vi "EncodeBase64.vi"(10 "string":string) -> (2 "base64 string":string)   [LabVIEW 2014]
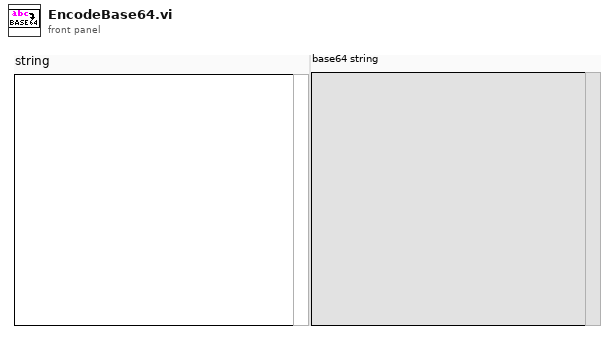
[diagram p1: front panel]
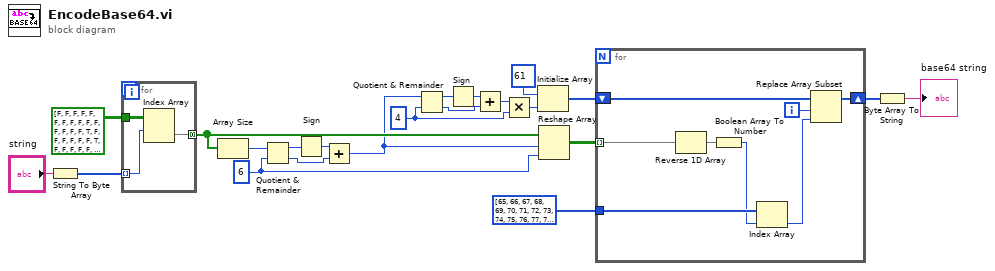
[diagram p0: block diagram]
diagram:
  w2 = 4 ("y")
  w19 = 6 ("y")
  n1 = String To Byte Array(string="string") -> (unsigned byte array=w11:u8[])
  n2 = for {
    tunnel: bool[][] [[FALSE, FALSE, FALSE, FALSE, FALSE, FALSE, FALSE, FALSE], [FALSE, FALSE, FALSE, FALSE, FALSE, FALSE, FALSE, TRUE], [FALSE, FALSE, FALSE, FALSE, FALSE, FALSE, TRUE, FALSE], [FALSE, FALSE, FALSE, FALSE, FALSE, FALSE, TRUE, TRUE], [FALSE, FALSE, FALSE, FALSE, FALSE, TRUE, FALSE, FALSE], [FALSE, FALSE, FALSE, FALSE, FALSE, TRUE, FALSE, TRUE], [FALSE, FALSE, FALSE, FALSE, FALSE, TRUE, TRUE, FALSE], [FALSE, FALSE, FALSE, FALSE, FALSE, TRUE, TRUE, TRUE], [FALSE, FALSE, FALSE, FALSE, TRUE, FALSE, FALSE, FALSE], [FALSE, FALSE, FALSE, FALSE, TRUE, FALSE, FALSE, TRUE], [FALSE, FALSE, FALSE, FALSE, TRUE, FALSE, TRUE, FALSE], [FALSE, FALSE, FALSE, FALSE, TRUE, FALSE, TRUE, TRUE], [FALSE, FALSE, FALSE, FALSE, TRUE, TRUE, FALSE, FALSE], [FALSE, FALSE, FALSE, FALSE, TRUE, TRUE, FALSE, TRUE], [FALSE, FALSE, FALSE, FALSE, TRUE, TRUE, TRUE, FALSE], [FALSE, FALSE, FALSE, FALSE, TRUE, TRUE, TRUE, TRUE], [FALSE, FALSE, FALSE, TRUE, FALSE, FALSE, FALSE, FALSE], [FALSE, FALSE, FALSE, TRUE, FALSE, FALSE, FALSE, TRUE], [FALSE, FALSE, FALSE, TRUE, FALSE, FALSE, TRUE, FALSE], [FALSE, FALSE, FALSE, TRUE, FALSE, FALSE, TRUE, TRUE], [FALSE, FALSE, FALSE, TRUE, FALSE, TRUE, FALSE, FALSE], [FALSE, FALSE, FALSE, TRUE, FALSE, TRUE, FALSE, TRUE], [FALSE, FALSE, FALSE, TRUE, FALSE, TRUE, TRUE, FALSE], [FALSE, FALSE, FALSE, TRUE, FALSE, TRUE, TRUE, TRUE], [FALSE, FALSE, FALSE, TRUE, TRUE, FALSE, FALSE, FALSE], [FALSE, FALSE, FALSE, TRUE, TRUE, FALSE, FALSE, TRUE], [FALSE, FALSE, FALSE, TRUE, TRUE, FALSE, TRUE, FALSE], [FALSE, FALSE, FALSE, TRUE, TRUE, FALSE, TRUE, TRUE], [FALSE, FALSE, FALSE, TRUE, TRUE, TRUE, FALSE, FALSE], [FALSE, FALSE, FALSE, TRUE, TRUE, TRUE, FALSE, TRUE], [FALSE, FALSE, FALSE, TRUE, TRUE, TRUE, TRUE, FALSE], [FALSE, FALSE, FALSE, TRUE, TRUE, TRUE, TRUE, TRUE], [FALSE, FALSE, TRUE, FALSE, FALSE, FALSE, FALSE, FALSE], [FALSE, FALSE, TRUE, FALSE, FALSE, FALSE, FALSE, TRUE], [FALSE, FALSE, TRUE, FALSE, FALSE, FALSE, TRUE, FALSE], [FALSE, FALSE, TRUE, FALSE, FALSE, FALSE, TRUE, TRUE], [FALSE, FALSE, TRUE, FALSE, FALSE, TRUE, FALSE, FALSE], [FALSE, FALSE, TRUE, FALSE, FALSE, TRUE, FALSE, TRUE], [FALSE, FALSE, TRUE, FALSE, FALSE, TRUE, TRUE, FALSE], [FALSE, FALSE, TRUE, FALSE, FALSE, TRUE, TRUE, TRUE], [FALSE, FALSE, TRUE, FALSE, TRUE, FALSE, FALSE, FALSE], [FALSE, FALSE, TRUE, FALSE, TRUE, FALSE, FALSE, TRUE], [FALSE, FALSE, TRUE, FALSE, TRUE, FALSE, TRUE, FALSE], [FALSE, FALSE, TRUE, FALSE, TRUE, FALSE, TRUE, TRUE], [FALSE, FALSE, TRUE, FALSE, TRUE, TRUE, FALSE, FALSE], [FALSE, FALSE, TRUE, FALSE, TRUE, TRUE, FALSE, TRUE], [FALSE, FALSE, TRUE, FALSE, TRUE, TRUE, TRUE, FALSE], [FALSE, FALSE, TRUE, FALSE, TRUE, TRUE, TRUE, TRUE], [FALSE, FALSE, TRUE, TRUE, FALSE, FALSE, FALSE, FALSE], [FALSE, FALSE, TRUE, TRUE, FALSE, FALSE, FALSE, TRUE], [FALSE, FALSE, TRUE, TRUE, FALSE, FALSE, TRUE, FALSE], [FALSE, FALSE, TRUE, TRUE, FALSE, FALSE, TRUE, TRUE], [FALSE, FALSE, TRUE, TRUE, FALSE, TRUE, FALSE, FALSE], [FALSE, FALSE, TRUE, TRUE, FALSE, TRUE, FALSE, TRUE], [FALSE, FALSE, TRUE, TRUE, FALSE, TRUE, TRUE, FALSE], [FALSE, FALSE, TRUE, TRUE, FALSE, TRUE, TRUE, TRUE], [FALSE, FALSE, TRUE, TRUE, TRUE, FALSE, FALSE, FALSE], [FALSE, FALSE, TRUE, TRUE, TRUE, FALSE, FALSE, TRUE], [FALSE, FALSE, TRUE, TRUE, TRUE, FALSE, TRUE, FALSE], [FALSE, FALSE, TRUE, TRUE, TRUE, FALSE, TRUE, TRUE], [FALSE, FALSE, TRUE, TRUE, TRUE, TRUE, FALSE, FALSE], [FALSE, FALSE, TRUE, TRUE, TRUE, TRUE, FALSE, TRUE], [FALSE, FALSE, TRUE, TRUE, TRUE, TRUE, TRUE, FALSE], [FALSE, FALSE, TRUE, TRUE, TRUE, TRUE, TRUE, TRUE], [FALSE, TRUE, FALSE, FALSE, FALSE, FALSE, FALSE, FALSE], [FALSE, TRUE, FALSE, FALSE, FALSE, FALSE, FALSE, TRUE], [FALSE, TRUE, FALSE, FALSE, FALSE, FALSE, TRUE, FALSE], [FALSE, TRUE, FALSE, FALSE, FALSE, FALSE, TRUE, TRUE], [FALSE, TRUE, FALSE, FALSE, FALSE, TRUE, FALSE, FALSE], [FALSE, TRUE, FALSE, FALSE, FALSE, TRUE, FALSE, TRUE], [FALSE, TRUE, FALSE, FALSE, FALSE, TRUE, TRUE, FALSE], [FALSE, TRUE, FALSE, FALSE, FALSE, TRUE, TRUE, TRUE], [FALSE, TRUE, FALSE, FALSE, TRUE, FALSE, FALSE, FALSE], [FALSE, TRUE, FALSE, FALSE, TRUE, FALSE, FALSE, TRUE], [FALSE, TRUE, FALSE, FALSE, TRUE, FALSE, TRUE, FALSE], [FALSE, TRUE, FALSE, FALSE, TRUE, FALSE, TRUE, TRUE], [FALSE, TRUE, FALSE, FALSE, TRUE, TRUE, FALSE, FALSE], [FALSE, TRUE, FALSE, FALSE, TRUE, TRUE, FALSE, TRUE], [FALSE, TRUE, FALSE, FALSE, TRUE, TRUE, TRUE, FALSE], [FALSE, TRUE, FALSE, FALSE, TRUE, TRUE, TRUE, TRUE], [FALSE, TRUE, FALSE, TRUE, FALSE, FALSE, FALSE, FALSE], [FALSE, TRUE, FALSE, TRUE, FALSE, FALSE, FALSE, TRUE], [FALSE, TRUE, FALSE, TRUE, FALSE, FALSE, TRUE, FALSE], [FALSE, TRUE, FALSE, TRUE, FALSE, FALSE, TRUE, TRUE], [FALSE, TRUE, FALSE, TRUE, FALSE, TRUE, FALSE, FALSE], [FALSE, TRUE, FALSE, TRUE, FALSE, TRUE, FALSE, TRUE], [FALSE, TRUE, FALSE, TRUE, FALSE, TRUE, TRUE, FALSE], [FALSE, TRUE, FALSE, TRUE, FALSE, TRUE, TRUE, TRUE], [FALSE, TRUE, FALSE, TRUE, TRUE, FALSE, FALSE, FALSE], [FALSE, TRUE, FALSE, TRUE, TRUE, FALSE, FALSE, TRUE], [FALSE, TRUE, FALSE, TRUE, TRUE, FALSE, TRUE, FALSE], [FALSE, TRUE, FALSE, TRUE, TRUE, FALSE, TRUE, TRUE], [FALSE, TRUE, FALSE, TRUE, TRUE, TRUE, FALSE, FALSE], [FALSE, TRUE, FALSE, TRUE, TRUE, TRUE, FALSE, TRUE], [FALSE, TRUE, FALSE, TRUE, TRUE, TRUE, TRUE, FALSE], [FALSE, TRUE, FALSE, TRUE, TRUE, TRUE, TRUE, TRUE], [FALSE, TRUE, TRUE, FALSE, FALSE, FALSE, FALSE, FALSE], [FALSE, TRUE, TRUE, FALSE, FALSE, FALSE, FALSE, TRUE], [FALSE, TRUE, TRUE, FALSE, FALSE, FALSE, TRUE, FALSE], [FALSE, TRUE, TRUE, FALSE, FALSE, FALSE, TRUE, TRUE], [FALSE, TRUE, TRUE, FALSE, FALSE, TRUE, FALSE, FALSE], [FALSE, TRUE, TRUE, FALSE, FALSE, TRUE, FALSE, TRUE], [FALSE, TRUE, TRUE, FALSE, FALSE, TRUE, TRUE, FALSE], [FALSE, TRUE, TRUE, FALSE, FALSE, TRUE, TRUE, TRUE], [FALSE, TRUE, TRUE, FALSE, TRUE, FALSE, FALSE, FALSE], [FALSE, TRUE, TRUE, FALSE, TRUE, FALSE, FALSE, TRUE], [FALSE, TRUE, TRUE, FALSE, TRUE, FALSE, TRUE, FALSE], [FALSE, TRUE, TRUE, FALSE, TRUE, FALSE, TRUE, TRUE], [FALSE, TRUE, TRUE, FALSE, TRUE, TRUE, FALSE, FALSE], [FALSE, TRUE, TRUE, FALSE, TRUE, TRUE, FALSE, TRUE], [FALSE, TRUE, TRUE, FALSE, TRUE, TRUE, TRUE, FALSE], [FALSE, TRUE, TRUE, FALSE, TRUE, TRUE, TRUE, TRUE], [FALSE, TRUE, TRUE, TRUE, FALSE, FALSE, FALSE, FALSE], [FALSE, TRUE, TRUE, TRUE, FALSE, FALSE, FALSE, TRUE], [FALSE, TRUE, TRUE, TRUE, FALSE, FALSE, TRUE, FALSE], [FALSE, TRUE, TRUE, TRUE, FALSE, FALSE, TRUE, TRUE], [FALSE, TRUE, TRUE, TRUE, FALSE, TRUE, FALSE, FALSE], [FALSE, TRUE, TRUE, TRUE, FALSE, TRUE, FALSE, TRUE], [FALSE, TRUE, TRUE, TRUE, FALSE, TRUE, TRUE, FALSE], [FALSE, TRUE, TRUE, TRUE, FALSE, TRUE, TRUE, TRUE], [FALSE, TRUE, TRUE, TRUE, TRUE, FALSE, FALSE, FALSE], [FALSE, TRUE, TRUE, TRUE, TRUE, FALSE, FALSE, TRUE], [FALSE, TRUE, TRUE, TRUE, TRUE, FALSE, TRUE, FALSE], [FALSE, TRUE, TRUE, TRUE, TRUE, FALSE, TRUE, TRUE], [FALSE, TRUE, TRUE, TRUE, TRUE, TRUE, FALSE, FALSE], [FALSE, TRUE, TRUE, TRUE, TRUE, TRUE, FALSE, TRUE], [FALSE, TRUE, TRUE, TRUE, TRUE, TRUE, TRUE, FALSE], [FALSE, TRUE, TRUE, TRUE, TRUE, TRUE, TRUE, TRUE], [TRUE, FALSE, FALSE, FALSE, FALSE, FALSE, FALSE, FALSE], [TRUE, FALSE, FALSE, FALSE, FALSE, FALSE, FALSE, TRUE], [TRUE, FALSE, FALSE, FALSE, FALSE, FALSE, TRUE, FALSE], [TRUE, FALSE, FALSE, FALSE, FALSE, FALSE, TRUE, TRUE], [TRUE, FALSE, FALSE, FALSE, FALSE, TRUE, FALSE, FALSE], [TRUE, FALSE, FALSE, FALSE, FALSE, TRUE, FALSE, TRUE], [TRUE, FALSE, FALSE, FALSE, FALSE, TRUE, TRUE, FALSE], [TRUE, FALSE, FALSE, FALSE, FALSE, TRUE, TRUE, TRUE], [TRUE, FALSE, FALSE, FALSE, TRUE, FALSE, FALSE, FALSE], [TRUE, FALSE, FALSE, FALSE, TRUE, FALSE, FALSE, TRUE], [TRUE, FALSE, FALSE, FALSE, TRUE, FALSE, TRUE, FALSE], [TRUE, FALSE, FALSE, FALSE, TRUE, FALSE, TRUE, TRUE], [TRUE, FALSE, FALSE, FALSE, TRUE, TRUE, FALSE, FALSE], [TRUE, FALSE, FALSE, FALSE, TRUE, TRUE, FALSE, TRUE], [TRUE, FALSE, FALSE, FALSE, TRUE, TRUE, TRUE, FALSE], [TRUE, FALSE, FALSE, FALSE, TRUE, TRUE, TRUE, TRUE], [TRUE, FALSE, FALSE, TRUE, FALSE, FALSE, FALSE, FALSE], [TRUE, FALSE, FALSE, TRUE, FALSE, FALSE, FALSE, TRUE], [TRUE, FALSE, FALSE, TRUE, FALSE, FALSE, TRUE, FALSE], [TRUE, FALSE, FALSE, TRUE, FALSE, FALSE, TRUE, TRUE], [TRUE, FALSE, FALSE, TRUE, FALSE, TRUE, FALSE, FALSE], [TRUE, FALSE, FALSE, TRUE, FALSE, TRUE, FALSE, TRUE], [TRUE, FALSE, FALSE, TRUE, FALSE, TRUE, TRUE, FALSE], [TRUE, FALSE, FALSE, TRUE, FALSE, TRUE, TRUE, TRUE], [TRUE, FALSE, FALSE, TRUE, TRUE, FALSE, FALSE, FALSE], [TRUE, FALSE, FALSE, TRUE, TRUE, FALSE, FALSE, TRUE], [TRUE, FALSE, FALSE, TRUE, TRUE, FALSE, TRUE, FALSE], [TRUE, FALSE, FALSE, TRUE, TRUE, FALSE, TRUE, TRUE], [TRUE, FALSE, FALSE, TRUE, TRUE, TRUE, FALSE, FALSE], [TRUE, FALSE, FALSE, TRUE, TRUE, TRUE, FALSE, TRUE], [TRUE, FALSE, FALSE, TRUE, TRUE, TRUE, TRUE, FALSE], [TRUE, FALSE, FALSE, TRUE, TRUE, TRUE, TRUE, TRUE], [TRUE, FALSE, TRUE, FALSE, FALSE, FALSE, FALSE, FALSE], [TRUE, FALSE, TRUE, FALSE, FALSE, FALSE, FALSE, TRUE], [TRUE, FALSE, TRUE, FALSE, FALSE, FALSE, TRUE, FALSE], [TRUE, FALSE, TRUE, FALSE, FALSE, FALSE, TRUE, TRUE], [TRUE, FALSE, TRUE, FALSE, FALSE, TRUE, FALSE, FALSE], [TRUE, FALSE, TRUE, FALSE, FALSE, TRUE, FALSE, TRUE], [TRUE, FALSE, TRUE, FALSE, FALSE, TRUE, TRUE, FALSE], [TRUE, FALSE, TRUE, FALSE, FALSE, TRUE, TRUE, TRUE], [TRUE, FALSE, TRUE, FALSE, TRUE, FALSE, FALSE, FALSE], [TRUE, FALSE, TRUE, FALSE, TRUE, FALSE, FALSE, TRUE], [TRUE, FALSE, TRUE, FALSE, TRUE, FALSE, TRUE, FALSE], [TRUE, FALSE, TRUE, FALSE, TRUE, FALSE, TRUE, TRUE], [TRUE, FALSE, TRUE, FALSE, TRUE, TRUE, FALSE, FALSE], [TRUE, FALSE, TRUE, FALSE, TRUE, TRUE, FALSE, TRUE], [TRUE, FALSE, TRUE, FALSE, TRUE, TRUE, TRUE, FALSE], [TRUE, FALSE, TRUE, FALSE, TRUE, TRUE, TRUE, TRUE], [TRUE, FALSE, TRUE, TRUE, FALSE, FALSE, FALSE, FALSE], [TRUE, FALSE, TRUE, TRUE, FALSE, FALSE, FALSE, TRUE], [TRUE, FALSE, TRUE, TRUE, FALSE, FALSE, TRUE, FALSE], [TRUE, FALSE, TRUE, TRUE, FALSE, FALSE, TRUE, TRUE], [TRUE, FALSE, TRUE, TRUE, FALSE, TRUE, FALSE, FALSE], [TRUE, FALSE, TRUE, TRUE, FALSE, TRUE, FALSE, TRUE], [TRUE, FALSE, TRUE, TRUE, FALSE, TRUE, TRUE, FALSE], [TRUE, FALSE, TRUE, TRUE, FALSE, TRUE, TRUE, TRUE], [TRUE, FALSE, TRUE, TRUE, TRUE, FALSE, FALSE, FALSE], [TRUE, FALSE, TRUE, TRUE, TRUE, FALSE, FALSE, TRUE], [TRUE, FALSE, TRUE, TRUE, TRUE, FALSE, TRUE, FALSE], [TRUE, FALSE, TRUE, TRUE, TRUE, FALSE, TRUE, TRUE], [TRUE, FALSE, TRUE, TRUE, TRUE, TRUE, FALSE, FALSE], [TRUE, FALSE, TRUE, TRUE, TRUE, TRUE, FALSE, TRUE], [TRUE, FALSE, TRUE, TRUE, TRUE, TRUE, TRUE, FALSE], [TRUE, FALSE, TRUE, TRUE, TRUE, TRUE, TRUE, TRUE], [TRUE, TRUE, FALSE, FALSE, FALSE, FALSE, FALSE, FALSE], [TRUE, TRUE, FALSE, FALSE, FALSE, FALSE, FALSE, TRUE], [TRUE, TRUE, FALSE, FALSE, FALSE, FALSE, TRUE, FALSE], [TRUE, TRUE, FALSE, FALSE, FALSE, FALSE, TRUE, TRUE], [TRUE, TRUE, FALSE, FALSE, FALSE, TRUE, FALSE, FALSE], [TRUE, TRUE, FALSE, FALSE, FALSE, TRUE, FALSE, TRUE], [TRUE, TRUE, FALSE, FALSE, FALSE, TRUE, TRUE, FALSE], [TRUE, TRUE, FALSE, FALSE, FALSE, TRUE, TRUE, TRUE], [TRUE, TRUE, FALSE, FALSE, TRUE, FALSE, FALSE, FALSE], [TRUE, TRUE, FALSE, FALSE, TRUE, FALSE, FALSE, TRUE], [TRUE, TRUE, FALSE, FALSE, TRUE, FALSE, TRUE, FALSE], [TRUE, TRUE, FALSE, FALSE, TRUE, FALSE, TRUE, TRUE], [TRUE, TRUE, FALSE, FALSE, TRUE, TRUE, FALSE, FALSE], [TRUE, TRUE, FALSE, FALSE, TRUE, TRUE, FALSE, TRUE], [TRUE, TRUE, FALSE, FALSE, TRUE, TRUE, TRUE, FALSE], [TRUE, TRUE, FALSE, FALSE, TRUE, TRUE, TRUE, TRUE], [TRUE, TRUE, FALSE, TRUE, FALSE, FALSE, FALSE, FALSE], [TRUE, TRUE, FALSE, TRUE, FALSE, FALSE, FALSE, TRUE], [TRUE, TRUE, FALSE, TRUE, FALSE, FALSE, TRUE, FALSE], [TRUE, TRUE, FALSE, TRUE, FALSE, FALSE, TRUE, TRUE], [TRUE, TRUE, FALSE, TRUE, FALSE, TRUE, FALSE, FALSE], [TRUE, TRUE, FALSE, TRUE, FALSE, TRUE, FALSE, TRUE], [TRUE, TRUE, FALSE, TRUE, FALSE, TRUE, TRUE, FALSE], [TRUE, TRUE, FALSE, TRUE, FALSE, TRUE, TRUE, TRUE], [TRUE, TRUE, FALSE, TRUE, TRUE, FALSE, FALSE, FALSE], [TRUE, TRUE, FALSE, TRUE, TRUE, FALSE, FALSE, TRUE], [TRUE, TRUE, FALSE, TRUE, TRUE, FALSE, TRUE, FALSE], [TRUE, TRUE, FALSE, TRUE, TRUE, FALSE, TRUE, TRUE], [TRUE, TRUE, FALSE, TRUE, TRUE, TRUE, FALSE, FALSE], [TRUE, TRUE, FALSE, TRUE, TRUE, TRUE, FALSE, TRUE], [TRUE, TRUE, FALSE, TRUE, TRUE, TRUE, TRUE, FALSE], [TRUE, TRUE, FALSE, TRUE, TRUE, TRUE, TRUE, TRUE], [TRUE, TRUE, TRUE, FALSE, FALSE, FALSE, FALSE, FALSE], [TRUE, TRUE, TRUE, FALSE, FALSE, FALSE, FALSE, TRUE], [TRUE, TRUE, TRUE, FALSE, FALSE, FALSE, TRUE, FALSE], [TRUE, TRUE, TRUE, FALSE, FALSE, FALSE, TRUE, TRUE], [TRUE, TRUE, TRUE, FALSE, FALSE, TRUE, FALSE, FALSE], [TRUE, TRUE, TRUE, FALSE, FALSE, TRUE, FALSE, TRUE], [TRUE, TRUE, TRUE, FALSE, FALSE, TRUE, TRUE, FALSE], [TRUE, TRUE, TRUE, FALSE, FALSE, TRUE, TRUE, TRUE], [TRUE, TRUE, TRUE, FALSE, TRUE, FALSE, FALSE, FALSE], [TRUE, TRUE, TRUE, FALSE, TRUE, FALSE, FALSE, TRUE], [TRUE, TRUE, TRUE, FALSE, TRUE, FALSE, TRUE, FALSE], [TRUE, TRUE, TRUE, FALSE, TRUE, FALSE, TRUE, TRUE], [TRUE, TRUE, TRUE, FALSE, TRUE, TRUE, FALSE, FALSE], [TRUE, TRUE, TRUE, FALSE, TRUE, TRUE, FALSE, TRUE], [TRUE, TRUE, TRUE, FALSE, TRUE, TRUE, TRUE, FALSE], [TRUE, TRUE, TRUE, FALSE, TRUE, TRUE, TRUE, TRUE], [TRUE, TRUE, TRUE, TRUE, FALSE, FALSE, FALSE, FALSE], [TRUE, TRUE, TRUE, TRUE, FALSE, FALSE, FALSE, TRUE], [TRUE, TRUE, TRUE, TRUE, FALSE, FALSE, TRUE, FALSE], [TRUE, TRUE, TRUE, TRUE, FALSE, FALSE, TRUE, TRUE], [TRUE, TRUE, TRUE, TRUE, FALSE, TRUE, FALSE, FALSE], [TRUE, TRUE, TRUE, TRUE, FALSE, TRUE, FALSE, TRUE], [TRUE, TRUE, TRUE, TRUE, FALSE, TRUE, TRUE, FALSE], [TRUE, TRUE, TRUE, TRUE, FALSE, TRUE, TRUE, TRUE], [TRUE, TRUE, TRUE, TRUE, TRUE, FALSE, FALSE, FALSE], [TRUE, TRUE, TRUE, TRUE, TRUE, FALSE, FALSE, TRUE], [TRUE, TRUE, TRUE, TRUE, TRUE, FALSE, TRUE, FALSE], [TRUE, TRUE, TRUE, TRUE, TRUE, FALSE, TRUE, TRUE], [TRUE, TRUE, TRUE, TRUE, TRUE, TRUE, FALSE, FALSE], [TRUE, TRUE, TRUE, TRUE, TRUE, TRUE, FALSE, TRUE], [TRUE, TRUE, TRUE, TRUE, TRUE, TRUE, TRUE, FALSE], [TRUE, TRUE, TRUE, TRUE, TRUE, TRUE, TRUE, TRUE]] ("Array") -> [w25]
    tunnel: w11 -> [w24] mode=indexing
    tunnel: [w23] -> w20 mode=concatenating
    n3 = Index Array(array=w25, index (row)=w24) -> (element=w23:bool[])  [unwired: 1 in]
  }
  n4 = Array Size(array=w20) -> (size(s)=w21:i32)
  n5 = Quotient & Remainder(x=w21, y=w19) -> (x-y*floor(x/y)=w10:i32, floor(x/y)=w8:i32)
  n6 = Sign(1:w10) -> (0:w9:i32)
  n7 = Add(x=w9, y=w8) -> (x+y=w3:i32)
  n8 = Quotient & Remainder(x=w3, y=w2) -> (x-y*floor(x/y)=w5:i32, floor(x/y)=w1:i32)
  n9 = Sign(1:w5) -> (0:w6:i32)
  n10 = Add(x=w6, y=w1) -> (x+y=w7:i32)
  n11 = Multiply(x=w7, y=w2) -> (x*y=w4:i32)
  n12 = Initialize Array(u8 61 ("y"), w4) -> (w13:u8[])
  n13 = Reshape Array(w20, w3, w19) -> (w18:bool[][])
  n14 = for {
    tunnel: w18 -> [w31] mode=indexing
    tunnel: u8[] [65, 66, 67, 68, 69, 70, 71, 72, 73, 74, 75, 76, 77, 78, 79, 80, 81, 82, 83, 84, 85, 86, 87, 88, 89, 90, 97, 98, 99, 100, 101, 102, 103, 104, 105, 106, 107, 108, 109, 110, 111, 112, 113, 114, 115, 116, 117, 118, 119, 120, 121, 122, 48, 49, 50, 51, 52, 53, 54, 55, 56, 57, 43, 47] ("unsigned byte array") -> [w33]
    shift-right: [w27] -> w12
    shift-left: w13 -> [w29]
    i -> [w26]
    n15 = Reverse 1D Array(array=w31) -> (reversed array=w30:bool[])
    n16 = Boolean Array To Number(Boolean array=w30) -> (number=w32:i32)
    n17 = Index Array(array=w33, index=w32) -> (element=w28:u8)
    n18 = Replace Array Subset(array=w29, new element=w28, index=w26) -> (w27:u8[])
  }
  n19 = Byte Array To String(unsigned byte array=w12) -> (string=→"base64 string":string)
